vi "ini_para.vi"(2 "End Position":sgl, 3 "Start Position":sgl, 4 "Step":sgl) -> (0 "Step Number":i32, 1 "Step":sgl)   [LabVIEW 2010]
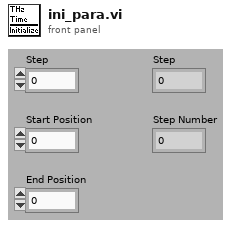
[diagram p1: front panel]
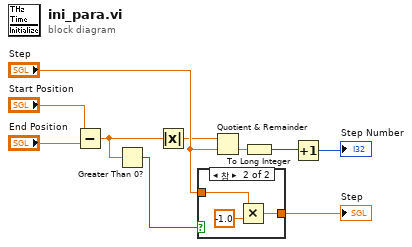
[diagram p0: block diagram]
diagram:
  n1 = Subtract(x="Start Position", y="End Position") -> (x-y=w7:sgl)
  n2 = Greater Than 0?(x=w7) -> (x > 0?=w8:bool)
  n3 = Absolute Value(x=w7) -> (abs(x)=w3:sgl)
  n4 = case shown="참" w8 {
    tunnel: "Step" -> [w11 w14]
    tunnel: [w11 w13] -> w10
    frame False {
    }
    frame True {
      n5 = Multiply(x=w14, y=sgl -1.0) -> (x*y=w13:sgl)
    }
  }
  "Step" <- w10
  n6 = Quotient & Remainder(x=w3, y="Step") -> (floor(x/y)=w6:sgl)  [unwired: 1 out]
  n7 = To Long Integer(number=w6) -> (32bit integer=w2:i32)
  n8 = Increment(x=w2) -> (x+1=→"Step Number":i32)
